vi "OSIPI OPCUA Server Tag Version.vi"(11 "Main Queue Cluster":T62) -> ()   [LabVIEW 2018]
uses:
  <vilib>/OPCUA/controls/NodeId.ctl
  <vilib>/OPCUA/controls/OPC UA Variable Node Refnum.ctl
  <vilib>/OPCUA/controls/OPC UA Server Refnum.ctl
  Drag and Drop/State Cluster.ctl
  support/Message Queue/Message Cluster.ctl
  Drag and Drop/Thumbnail Cluster.ctl
  Drag and Drop/Object Cluster.ctl
  <vilib>/Utility/miscctls.llb/LVRectTypeDef.ctl
  Drag and Drop/Object Type Enum.ctl
  <vilib>/Utility/miscctls.llb/LVPositionTypeDef.ctl
  Config Module/Controls/Main Config Cluster.ctl
  OPC Module Config.ctl
  Scale Module Folder/Measure Instrument/State Enum.ctl
  <vilib>/Utility/miscctls.llb/LVPoint32TypeDef.ctl
  OPC Settings.ctl
  Variable Data Cluster.ctl
  <vilib>/OPCUA/controls/OPC UA StatusCode.ctl
  <vilib>/OPCUA/controls/Subscription ID.ctl
  <vilib>/OPCUA/controls/OPC UA Client Refnum.ctl
  <vilib>/OPCUA/controls/Subscription Data Change.ctl
  <vilib>/OPCUA/controls/Data Type.ctl
  Feed Module/Controls/Feed Module Config Cluster.ctl
  Feed Module/Controls/Feed Module Settings Cluster.ctl
  Ismatec ISM 831C/Controls/Ismatech Settings Cluster.ctl
  Masterflex 7550-30/Controls/Settings Cluster.ctl
  Mettler Toledo/Controls/Settings Cluster.ctl
  Bronkhorst M13 Flow Meter/Settings Cluster.ctl
  Measure Instrument/PID 2 Parameters Cluster.ctl
  Measure Instrument/PID Input Enum.ctl
  Measure Instrument/PID 2 Output Enum.ctl
  Tacmina QI/Tacmina QI DAQ Setting.ctl
  KNF Pump/Settings Cluster plus SIMDOS.ctl
  ASIA Pump/Pump Settings.ctl
  VICI M50 Party Mode/Settings Cluster.ctl
  FLOM Pump/Settings Cluster.ctl
  SSI PR Class/SSI PR Settings Cluster.ctl
  TT Module/Controls/TT Module Config Cluster.ctl
  Acquisition/Hardware Configuration.ctl
  Acquisition/Task Cluster.ctl
  PT Module/Controls/PT Module Config Cluster.ctl
  Scale Module Folder/Feed Module/Controls/Scale Module Config Cluster.ctl
  Scale Module Folder/Feed Module/Controls/Scale Module Settings Cluster.ctl
  Pump Module Folder/Pump Module Config Cluster.ctl
  Pump Module Folder/Pump Module Settings Cluster.ctl
  LabJack Module/Controls/U3 Module Config Cluster.ctl
  Decoration Module/Decoration Module Config Cluster.ctl
  Flow Module Folder/Feed Module/Controls/Flow Module Config Cluster.ctl
  Flow Module Folder/Feed Module/Controls/Flow Module Settings Cluster.ctl
  TCU Module/TCU Module Folder/TCU Module Config Cluster.ctl
  TCU Module/TCU Module Folder/TCU Module Settings Cluster.ctl
  TCU Module/TCU Module Folder/Measure Instrument/Output Devices.ctl
  Huber TCU/Huber Settings.ctl
  Lauda Integral XT-150 TCU/Lauda Settings.ctl
  Julabo Type 1 TCU/Julabo Type 1 TCU Folder/Julabo FP-50 Settings.ctl
  Huber Unistat 410 TCU/Huber Unistat 410 Settings.ctl
  D-O Module Folder/Not Sure Where this is Used.ctl
  Sequencing/Squence Control.ctl
  D-O Module Folder/D-O Module Config Cluster.ctl
  D-O Module Folder/Valve Clusters.ctl
  D-O Module Folder/D-O Module Settings Cluster.ctl
  D-O Module Folder/D-O Device Settings Cluster.ctl
  VICI Electronic Actuator/VICI Electronic Actuator Settings.ctl
  Pressure Regulator Control Module/Pressure Regulator/Controls/4-20mA Module Config Cluster.ctl
  Pressure Regulator Control Module/Pressure Regulator/Controls/4-20mA Module Settings Cluster.ctl
  Pressure Transmitter/Pressure Transmitter Device Settings.ctl
  Pressure Reg Module/Pressure Regulator Device Settings.ctl
  <vilib>/OPCUA/controls/Supported Security Policies.ctl
  Tag VIs/Tag FGV Operation Enum.ctl
  <vilib>/OPCUA/server/Write Double.vi
  <vilib>/OPCUA/NI OPC UA Server.lvlib
  Shared Variables/Dynamic Shared Variables.lvlib
  support/Message Queue/Message Queue.lvlib
  support/Message Queue/Enqueue Message (Single).vi
  TT Module/TT Module.lvlib
  Masterflex 7550-30/Masterflex 7550-30.lvlib
  Ismatec ISM 831C/Ismatec ISM 831C.lvlib
  Tacmina QI/Tacmina QI.lvlib
  KNF Pump/KNF SIMDOS.lvlib
  VICI M50 Party Mode/VICI M6 M50 Party Mode.lvlib
  FLOM Pump/FLOM Pump.lvlib
  ASIA Pump.lvlib
  Mettler Toledo/Mettler Toledo.lvlib
  Bronkhorst M13 Flow Meter/Bronkhorst M13 Flow Meter.lvlib
  SSI PR Class/SSI PR Pump.lvlib
  Feed Module/Feed Module.lvlib
  DAQ/DAQ.lvlib
  PT Module/PT Module.lvlib
  Scale Module Folder/Scale Module.lvlib
  Pump Module Folder/Pump Module.lvlib
  LabJack Module/U3 Module.lvlib
  Flow Module Folder/Flow Module.lvlib
  Huber TCU/Huber Ministat 230 TCU.lvlib
  Lauda Integral XT-150 TCU/Lauda TCU.lvlib
  Julabo Type 1 TCU/Julabo Type 1 TCU Folder/Julabo Type FP-50 TCU.lvlib
  Huber Unistat 410 TCU/Huber Unistat 410 TCU.lvlib
  TCU Module/TCU Module Folder/TCU Module.lvlib
  Sequencing/Sequencing Library.lvlib
  D-O Module Folder/D-O Module.lvlib
  D-O Module Folder/DIO Valve/VICI Electronic Actuator.lvlib
  Pressure Transmitter/Pressure Transmitter Library.lvlib
  Pressure Reg Module/Pressure Regulator Library.lvlib
  Pressure Regulator Control Module/Pressure Regulator/4-20mA Module.lvlib
  OPC UA.lvlib
  Scale Module Folder/Measure Instrument/Scale Module Engine.lvlib
  Config Module/Config Module.lvlib
  Drag and Drop/Drag and Drop.lvlib
panel:
  in  "?":T1={"VI refs"=[], "Queues"=[], "[Thumbnails]"=[], "Drag Object Idx"=0, "[Objects]"=[], "Active Object"=0, "Drop Offset"={"Left"=0, "Top"=0}, "Process Name"="", "Main Config"={"OPC Module Configs"=[], "Feed Module Configs"=[], "Log File Path"=path "", "TT Module Configs"=[], "DAQ Config"={"Tasks"=[]}, "PT Module Configs"=[], "Scale Module Configs"=[], "Pump Module Configs"=[], "U3 Module Configs"=[{"GUID"="", "Drop Coords"={"Horizontal"=0, "Vertical"=0}, "AI Channel Number"=enum."Default", "Process Name"="", "Input Channel Numeric Alarm Settings"=[]}], "Decoration Module Configs"=[], "Flow Module Configs"=[], "TCU Module Configs"=[], "Steps"=[], "Abort"=FALSE, "DO Module Configs"=[], "PR Module Configs"=[], "Cycle Period"=0.0}, "Campaign Filepath"=path "", "Config Changed?"=FALSE} {"Main Config"."PR Module Configs"."Settings"."PID 2 Parameters"."output range"."output low" format="%.2f"; "Main Config"."PR Module Configs"."Settings"."PID 2 Parameters"."output range"."output high" min=0.0 max=100.0 format="%.2f"; "Main Config"."PR Module Configs"."Settings"."PID 2 Parameters"."PID gains"."derivative time (Td, min)" format="%.3f"; "Main Config"."PR Module Configs"."Settings"."PID 2 Parameters"."PID gains"."integral time (Ti, min)" format="%.3f"; "Main Config"."PR Module Configs"."Settings"."PID 2 Parameters"."PID gains"."proportional gain (Kc)" format="%.3f"; "Main Config"."Steps"."Control" items=["Pump %", "Setpoint"]; "Main Config"."TCU Module Configs"."Settings"."Julabo FP-50 Settings"."Pump Power" min=0 max=8 step=1; "Main Config"."TCU Module Configs"."Settings"."Lauda Settings"."Pump Power" min=0 max=8 step=1; "Main Config"."Pump Module Configs"."Settings"."ASIA Pump C"."channel" min=0 max=1 step=1; "Main Config"."Pump Module Configs"."Settings"."Masterflex"."Pump Number" min=1.0 max=20.0 step=1.0; "Main Config"."Pump Module Configs"."Settings"."Ismatech"."Pump Number" min=1.0 max=20.0 step=1.0; "Main Config"."Feed Module Configs"."Settings"."output range"."output low" min=0.0 max=100.0 format="%.2f"; "Main Config"."Feed Module Configs"."Settings"."output range"."output high" format="%.2f"; "Main Config"."Feed Module Configs"."Settings"."PID 2 Parameters"."PID gains"."derivative time (Td, min)" format="%.3f"; "Main Config"."Feed Module Configs"."Settings"."PID 2 Parameters"."PID gains"."integral time (Ti, min)" format="%.3f"; "Main Config"."Feed Module Configs"."Settings"."PID 2 Parameters"."PID gains"."proportional gain (Kc)" format="%.3f"; "Main Config"."Feed Module Configs"."Settings"."ASIA Pump C"."channel" min=0 max=1 step=1; "Main Config"."Feed Module Configs"."Settings"."Ismatech"."Pump Number" min=1.0 max=20.0 step=1.0; "Main Config"."Feed Module Configs"."Settings"."Masterflex"."Pump Number" min=1.0 max=20.0 step=1.0}
  in  "supported security policies (None)":T63={"None"=TRUE, "Sign with Basic128Rsa15"=TRUE, "Sign and Encrypt with Basic128Rsa15"=TRUE, "Sign with Basic256"=TRUE, "Sign and Encrypt with Basic256"=TRUE}
  out "Tag Values":dbl[](array[numeric])
  out "Tag Names":string[](array[string])
  out "Array":T65(array[cluster])
  out "OPC UA server refnum out":T66
  out "Array 2":T14[](array[typedef]) items=["Good"=0, "Good_SubscriptionTransferred"=2949120, "Good_CompletesAsynchronously"=3014656, "Good_Overload"=3080192, "Good_Clamped"=3145728, "Good_LocalOverride"=9830400, "Good_EntryInserted"=10616832, "Good_EntryReplaced"=10682368, "Good_NoData"=10813440, "Good_MoreData"=10878976, "Good_CommunicationEvent"=10944512, "Good_ShutdownEvent"=11010048, "Good_CallAgain"=11075584, "Good_NonCriticalTimeout"=11141120, "Good_ResultsMayBeIncomplete"=12189696, "Good_DataIgnored"=14221312, "Uncertain"=1073741824, "Uncertain_ReferenceOutOfServer"=1080819712, "Uncertain_NoCommunicationLastUsableValue"=1083113472, "Uncertain_LastUsableValue"=1083179008, "Uncertain_SubstituteValue"=1083244544, "Uncertain_InitialValue"=1083310080, "Uncertain_SensorNotAccurate"=1083375616, "Uncertain_EngineeringUnitsExceeded"=1083441152, "Uncertain_SubNormal"=1083506688, "Uncertain_DataSubNormal"=1084489728, "Uncertain_ReferenceNotDeleted"=1086062592, "Uncertain_NotAllNodesAvailable"=1086324736, "Bad"=2147483648, "Bad_UnexpectedError"=2147549184, "Bad_InternalError"=2147614720, "Bad_OutOfMemory"=2147680256, "Bad_ResourceUnavailable"=2147745792, "Bad_CommunicationError"=2147811328, "Bad_EncodingError"=2147876864, "Bad_DecodingError"=2147942400, "Bad_EncodingLimitsExceeded"=2148007936, "Bad_UnknownResponse"=2148073472, "Bad_Timeout"=2148139008, "Bad_ServiceUnsupported"=2148204544, "Bad_Shutdown"=2148270080, "Bad_ServerNotConnected"=2148335616, "Bad_ServerHalted"=2148401152, "Bad_NothingToDo"=2148466688, "Bad_TooManyOperations"=2148532224, "Bad_DataTypeIdUnknown"=2148597760, "Bad_CertificateInvalid"=2148663296, "Bad_SecurityChecksFailed"=2148728832, "Bad_CertificateTimeInvalid"=2148794368, "Bad_CertificateIssuerTimeInvalid"=2148859904, "Bad_CertificateHostNameInvalid"=2148925440, "Bad_CertificateUriInvalid"=2148990976, "Bad_CertificateUseNotAllowed"=2149056512, "Bad_CertificateIssuerUseNotAllowed"=2149122048, "Bad_CertificateUntrusted"=2149187584, "Bad_CertificateRevocationUnknown"=2149253120, "Bad_CertificateIssuerRevocationUnknown"=2149318656, "Bad_CertificateRevoked"=2149384192, "Bad_CertificateIssuerRevoked"=2149449728, "Bad_UserAccessDenied"=2149515264, "Bad_IdentityTokenInvalid"=2149580800, "Bad_IdentityTokenRejected"=2149646336, "Bad_SecureChannelIdInvalid"=2149711872, "Bad_InvalidTimestamp"=2149777408, "Bad_NonceInvalid"=2149842944, "Bad_SessionIdInvalid"=2149908480, "Bad_SessionClosed"=2149974016, "Bad_SessionNotActivated"=2150039552, "Bad_SubscriptionIdInvalid"=2150105088, "Bad_RequestHeaderInvalid"=2150236160, "Bad_TimestampsToReturnInvalid"=2150301696, "Bad_RequestCancelledByClient"=2150367232, "Bad_NoCommunication"=2150694912, "Bad_WaitingForInitialData"=2150760448, "Bad_NodeIdInvalid"=2150825984, "Bad_NodeIdUnknown"=2150891520, "Bad_AttributeIdInvalid"=2150957056, "Bad_IndexRangeInvalid"=2151022592, "Bad_IndexRangeNoData"=2151088128, "Bad_DataEncodingInvalid"=2151153664, "Bad_DataEncodingUnsupported"=2151219200, "Bad_NotReadable"=2151284736, "Bad_NotWritable"=2151350272, "Bad_OutOfRange"=2151415808, "Bad_NotSupported"=2151481344, "Bad_NotFound"=2151546880, "Bad_ObjectDeleted"=2151612416, "Bad_NotImplemented"=2151677952, "Bad_MonitoringModeInvalid"=2151743488, "Bad_MonitoredItemIdInvalid"=2151809024, "Bad_MonitoredItemFilterInvalid"=2151874560, "Bad_MonitoredItemFilterUnsupported"=2151940096, "Bad_FilterNotAllowed"=2152005632, "Bad_StructureMissing"=2152071168, "Bad_EventFilterInvalid"=2152136704, "Bad_ContentFilterInvalid"=2152202240, "Bad_FilterOperandInvalid"=2152267776, "Bad_ContinuationPointInvalid"=2152333312, "Bad_NoContinuationPoints"=2152398848, "Bad_ReferenceTypeIdInvalid"=2152464384, "Bad_BrowseDirectionInvalid"=2152529920, "Bad_NodeNotInView"=2152595456, "Bad_ServerUriInvalid"=2152660992, "Bad_ServerNameMissing"=2152726528, "Bad_DiscoveryUrlMissing"=2152792064, "Bad_SempahoreFileMissing"=2152857600, "Bad_RequestTypeInvalid"=2152923136, "Bad_SecurityModeRejected"=2152988672, "Bad_SecurityPolicyRejected"=2153054208, "Bad_TooManySessions"=2153119744, "Bad_UserSignatureInvalid"=2153185280, "Bad_ApplicationSignatureInvalid"=2153250816, "Bad_NoValidCertificates"=2153316352, "Bad_RequestCancelledByRequest"=2153381888, "Bad_ParentNodeIdInvalid"=2153447424, "Bad_ReferenceNotAllowed"=2153512960, "Bad_NodeIdRejected"=2153578496, "Bad_NodeIdExists"=2153644032, "Bad_NodeClassInvalid"=2153709568, "Bad_BrowseNameInvalid"=2153775104, "Bad_BrowseNameDuplicated"=2153840640, "Bad_NodeAttributesInvalid"=2153906176, "Bad_TypeDefinitionInvalid"=2153971712, "Bad_SourceNodeIdInvalid"=2154037248, "Bad_TargetNodeIdInvalid"=2154102784, "Bad_DuplicateReferenceNotAllowed"=2154168320, "Bad_InvalidSelfReference"=2154233856, "Bad_ReferenceLocalOnly"=2154299392, "Bad_NoDeleteRights"=2154364928, "Bad_ServerIndexInvalid"=2154430464, "Bad_ViewIdUnknown"=2154496000, "Bad_TooManyMatches"=2154627072, "Bad_QueryTooComplex"=2154692608, "Bad_NoMatch"=2154758144, "Bad_MaxAgeInvalid"=2154823680, "Bad_HistoryOperationInvalid"=2154889216, "Bad_HistoryOperationUnsupported"=2154954752, "Bad_WriteNotSupported"=2155020288, "Bad_TypeMismatch"=2155085824, "Bad_MethodInvalid"=2155151360, "Bad_ArgumentsMissing"=2155216896, "Bad_TooManySubscriptions"=2155282432, "Bad_TooManyPublishRequests"=2155347968, "Bad_NoSubscription"=2155413504, "Bad_SequenceNumberUnknown"=2155479040, "Bad_MessageNotAvailable"=2155544576, "Bad_InsufficientClientProfile"=2155610112, "Bad_TcpServerTooBusy"=2155675648, "Bad_TcpMessageTypeInvalid"=2155741184, "Bad_TcpSecureChannelUnknown"=2155806720, "Bad_TcpMessageTooLarge"=2155872256, "Bad_TcpNotEnoughResources"=2155937792, "Bad_TcpInternalError"=2156003328, "Bad_TcpEndpointUrlInvalid"=2156068864, "Bad_RequestInterrupted"=2156134400, "Bad_RequestTimeout"=2156199936, "Bad_SecureChannelClosed"=2156265472, "Bad_SecureChannelTokenUnknown"=2156331008, "Bad_SequenceNumberInvalid"=2156396544, "Bad_ConfigurationError"=2156462080, "Bad_NotConnected"=2156527616, "Bad_DeviceFailure"=2156593152, "Bad_SensorFailure"=2156658688, "Bad_OutOfService"=2156724224, "Bad_DeadbandFilterInvalid"=2156789760, "Bad_RefreshInProgress"=2157379584, "Bad_ConditionAlreadyDisabled"=2157445120, "Bad_ConditionDisabled"=2157510656, "Bad_EventIdUnknown"=2157576192, "Bad_NoData"=2157641728, "Bad_DataLost"=2157772800, "Bad_DataUnavailable"=2157838336, "Bad_EntryExists"=2157903872, "Bad_NoEntryExists"=2157969408, "Bad_TimestampNotSupported"=2158034944, "Bad_InvalidArgument"=2158690304, "Bad_ConnectionRejected"=2158755840, "Bad_Disconnect"=2158821376, "Bad_ConnectionClosed"=2158886912, "Bad_InvalidState"=2158952448, "Bad_EndOfStream"=2159017984, "Bad_NoDataAvailable"=2159083520, "Bad_WaitingForResponse"=2159149056, "Bad_OperationAbandoned"=2159214592, "Bad_ExpectedStreamToBlock"=2159280128, "Bad_WouldBlock"=2159345664, "Bad_SyntaxError"=2159411200, "Bad_MaxConnectionsReached"=2159476736, "Bad_RequestTooLarge"=2159542272, "Bad_ResponseTooLarge"=2159607808, "Bad_EventNotAcknowledgeable"=2159738880, "Bad_InvalidTimestampArgument"=2159869952, "Bad_ProtocolVersionUnsupported"=2159935488, "Bad_StateNotActive"=2160001024, "Bad_FilterOperatorInvalid"=2160132096, "Bad_FilterOperatorUnsupported"=2160197632, "Bad_FilterOperandCountMismatch"=2160263168, "Bad_FilterElementInvalid"=2160328704, "Bad_FilterLiteralInvalid"=2160394240, "Bad_IdentityChangeNotSupported"=2160459776, "Bad_NotTypeDefinition"=2160590848, "Bad_ViewTimestampInvalid"=2160656384, "Bad_ViewParameterMismatch"=2160721920, "Bad_ViewVersionInvalid"=2160787456, "Bad_ConditionAlreadyEnabled"=2160852992, "Bad_DialogNotActive"=2160918528, "Bad_DialogResponseInvalid"=2160984064, "Bad_ConditionBranchAlreadyAcked"=2161049600, "Bad_ConditionBranchAlreadyConfirmed"=2161115136, "Bad_ConditionAlreadyShelved"=2161180672, "Bad_ConditionNotShelved"=2161246208, "Bad_ShelvingTimeOutOfRange"=2161311744, "Bad_AggregateListMismatch"=2161377280, "Bad_AggregateNotSupported"=2161442816, "Bad_AggregateInvalidInputs"=2161508352, "Bad_BoundNotFound"=2161573888, "Bad_BoundNotSupported"=2161639424, "Bad_AggregateConfigurationRejected"=2161770496, "Bad_TooManyMonitoredItems"=2161836032]
  out "server endpoint URL":string
  in  "?":T1 {"Main Config"."PR Module Configs"."Settings"."PID 2 Parameters"."output range"."output low" format="%.2f"; "Main Config"."PR Module Configs"."Settings"."PID 2 Parameters"."output range"."output high" min=0.0 max=100.0 format="%.2f"; "Main Config"."PR Module Configs"."Settings"."PID 2 Parameters"."PID gains"."derivative time (Td, min)" format="%.3f"; "Main Config"."PR Module Configs"."Settings"."PID 2 Parameters"."PID gains"."integral time (Ti, min)" format="%.3f"; "Main Config"."PR Module Configs"."Settings"."PID 2 Parameters"."PID gains"."proportional gain (Kc)" format="%.3f"; "Main Config"."Steps"."Control" items=["Pump %", "Setpoint"]; "Main Config"."TCU Module Configs"."Settings"."Julabo FP-50 Settings"."Pump Power" min=0 max=8 step=1; "Main Config"."TCU Module Configs"."Settings"."Lauda Settings"."Pump Power" min=0 max=8 step=1; "Main Config"."Pump Module Configs"."Settings"."ASIA Pump C"."channel" min=0 max=1 step=1; "Main Config"."Pump Module Configs"."Settings"."Masterflex"."Pump Number" min=1.0 max=20.0 step=1.0; "Main Config"."Pump Module Configs"."Settings"."Ismatech"."Pump Number" min=1.0 max=20.0 step=1.0; "Main Config"."Feed Module Configs"."Settings"."output range"."output low" min=0.0 max=100.0 format="%.2f"; "Main Config"."Feed Module Configs"."Settings"."output range"."output high" format="%.2f"; "Main Config"."Feed Module Configs"."Settings"."PID 2 Parameters"."PID gains"."derivative time (Td, min)" format="%.3f"; "Main Config"."Feed Module Configs"."Settings"."PID 2 Parameters"."PID gains"."integral time (Ti, min)" format="%.3f"; "Main Config"."Feed Module Configs"."Settings"."PID 2 Parameters"."PID gains"."proportional gain (Kc)" format="%.3f"; "Main Config"."Feed Module Configs"."Settings"."ASIA Pump C"."channel" min=0 max=1 step=1; "Main Config"."Feed Module Configs"."Settings"."Ismatech"."Pump Number" min=1.0 max=20.0 step=1.0; "Main Config"."Feed Module Configs"."Settings"."Masterflex"."Pump Number" min=1.0 max=20.0 step=1.0}
  out "OPC UA server refnum out 3":T66
  out "Array 3":T65(array[cluster])
  # "Instrument Settings"
  # "Instrument Settings"
  # "Output Instruments"
  # "Flow Meter Settings"
  # "Output Instruments"
  # "Scale Settings"
  # "Output Instruments"
  # "Input Instruments"
  # "Instrument Settings"
  # "Instrument Settings"
  # "Output Instruments"
  # "Flow Meter Settings"
  # "Output Instruments"
  # "Scale Settings"
  # "Output Instruments"
  # "Input Instruments"
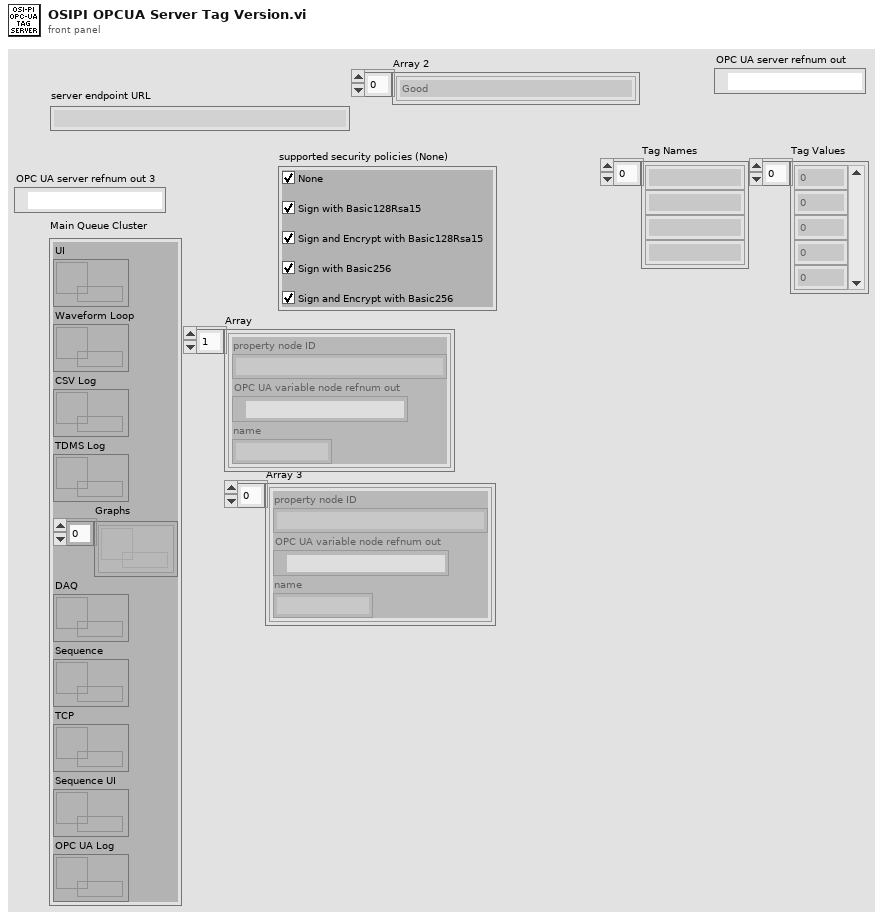
[diagram p1: front panel]
types:
  T1 = typedef "Drag and Drop.lvlib/State Cluster.ctl" = cluster{"VI refs":refnum<vi>[], "Queues":refnum<queue>[], "[Thumbnails]":T2[], "Drag Object Idx":i32, "[Objects]":T3[], "Active Object":i32, "Drop Offset":T6, "Process Name":string, "Main Config":T7, "Campaign Filepath":path, "Config Changed?":bool}
  T2 = typedef "Thumbnail Cluster.ctl" = cluster{"Path":path, "Rectangle":cluster{"left":i16, "top":i16, "right":i16, "bottom":i16}}
  T3 = typedef "Object Cluster.ctl" = cluster{"BMP Path":path, "Anchor Position":cluster{"X":i32, "Y":i32}, "Hot Spot":T4, "Type":T5, "Parameters":variant}
  T4 = typedef "LVRectTypeDef.ctl" = cluster{"Left":i16, "Top":i16, "Right":i16, "Bottom":i16}
  T5 = typedef "Object Type Enum.ctl" = enum16{"Icon", "Line", "Text", "Feed Module"}
  T6 = typedef "LVPositionTypeDef.ctl" = cluster{"Left":i32, "Top":i32}
  T7 = typedef "Config Module.lvlib/Main Config Cluster.ctl" = cluster{"OPC Module Configs":T8[], "Feed Module Configs":T17[], "Log File Path":path, "TT Module Configs":T32[], "DAQ Config":T33, "PT Module Configs":T35[], "Scale Module Configs":T36[], "Pump Module Configs":T38[], "U3 Module Configs":T40[], "Decoration Module Configs":T41[], "Flow Module Configs":T42[], "TCU Module Configs":T44[], "Steps":T51, "Abort":bool, "DO Module Configs":T53[], "PR Module Configs":T58[], "Cycle Period":dbl}
  T8 = typedef "OPC UA.lvlib/OPC Module Config.ctl" = cluster{"State":T9, "GUID":string, "Drop Coords":T10, "Configuration":T11, "First Iteration":bool, "Data":cluster{"Object Name":string, "Variable Array":T12[]}[], "Process Name":string, "Load Count":i32, "Log Started":bool, "subscription ID out":T15, "OPC UA client refnum out":T16, "Event Registration Refnum":refnum<event-registration>, "Start Time":timestamp, "Current Time":timestamp}
  T9 = typedef "Scale Module.lvlib/Scale Module Engine.lvlib/State Enum.ctl" = enum16{"Measuring", "Idle"}
  T10 = typedef "LVPoint32TypeDef.ctl" = cluster{"Horizontal":i32, "Vertical":i32}
  T11 = typedef "OPC UA.lvlib/OPC Settings.ctl" = cluster{"Cycle Period":dbl, "server endpoint URL":string, "security policy":cluster{"message mode":enum16{"None", "Sign", "Sign and Encrypt"}, "security":enum16{"Basic256", "Basic128Rsa15"}}, "Trust Any Server":bool}
  T12 = typedef "OPC UA.lvlib/Variable Data Cluster.ctl" = cluster{"node ID":T13, "browse name":string, "status":T14, "timestamp":timestamp, "value ":variant}
  T13 = typedef "NodeId.ctl" = string
  T14 = typedef "OPC UA StatusCode.ctl" = u32
  T15 = typedef "Subscription ID.ctl" = u32
  T16 = typedef "OPC UA Client Refnum.ctl" = refnum<k21>
  T17 = typedef "Feed Module.lvlib/Feed Module Config Cluster.ctl" = cluster{"GUID":string, "Drop Coords":T10, "Process Name":string, "Settings":T18, "Settings Load Count":i32, "OP Load Count":i32}
  T18 = typedef "Feed Module.lvlib/Feed Module Settings Cluster.ctl" = cluster{"Cycle Period":dbl, "Ismatech":T19, "Masterflex":T20, "Mettler":T21, "Bronkhorst M13 Flow Meter":T22, "PID 2 Parameters":T23, "Manual Entry":dbl, "Auto?":bool, "output range":cluster{"output high":dbl, "output low":dbl}, "Bronkhorst M14":T21, "Tacmina Settings":T26, "KNF SIMDOS Settings":T27, "ASIA Pump C":T28, "VICI Settings":T29, "FLOM Settings":T30, "SSI PR Settings":T31}
  T19 = typedef "Ismatec ISM 831C.lvlib/Ismatech Settings Cluster.ctl" = cluster{"VISA resource name":refnum<visa-resource-name>, "Simulated?":bool, "Pump Number":dbl, "Reverse?":bool}
  T20 = typedef "Masterflex 7550-30.lvlib/Settings Cluster.ctl" = cluster{"VISA resource name":refnum<visa-resource-name>, "Simulated?":bool, "Pump Number":dbl, "Reverse?":bool}
  T21 = typedef "Mettler Toledo.lvlib/Settings Cluster.ctl" = cluster{"VISA resource name":refnum<visa-resource-name>, "Simulated?":bool}
  T22 = typedef "Bronkhorst M13 Flow Meter.lvlib/Settings Cluster.ctl" = cluster{"VISA resource name":refnum<visa-resource-name>, "Simulated?":bool}
  T23 = typedef "PID 2 Parameters Cluster.ctl" = cluster{"Input Device":T24, "Output Device":T25, "Setpoint":dbl, "PID gains":cluster{"proportional gain (Kc)":dbl, "integral time (Ti, min)":dbl, "derivative time (Td, min)":dbl}}
  T24 = typedef "PID Input Enum.ctl" = enum16{"Default", "Bronkhorst M13", "Bronkhorst M14", "Scale Rate of Change"}
  T25 = typedef "PID 2 Output Enum.ctl" = enum16{"Default", "Ismatec ISM 831C", "Masterflex 7550-30", "VICI", "Tacmina QI", "KNF SIMDOS", "ASIA Type C", "FLOM UI-22-11", "SSI PR"}
  T26 = typedef "Tacmina QI.lvlib/Tacmina QI DAQ Setting.ctl" = cluster{"Analog DAQ Task":refnum<k21>, "Digital DAQ Task":refnum<k21>}
  T27 = typedef "KNF SIMDOS.lvlib/Settings Cluster plus SIMDOS.ctl" = cluster{"VISA resource name":refnum<visa-resource-name>, "Simulated?":bool}
  T28 = typedef "ASIA Pump.lvlib/Pump Settings.ctl" = cluster{"ASIA Pump #":i32, "channel":i32, "Simulated":bool}
  T29 = typedef "VICI M6 M50 Party Mode.lvlib/Settings Cluster.ctl" = cluster{"VISA resource name":refnum<visa-resource-name>, "Simulated?":bool, "Pump Letter":string, "Reverse?":bool}
  T30 = typedef "FLOM Pump.lvlib/Settings Cluster.ctl" = cluster{"VISA resource name":refnum<visa-resource-name>, "Simulated?":bool, "Pump Number":dbl}
  T31 = typedef "SSI PR Pump.lvlib/SSI PR Settings Cluster.ctl" = cluster{"VISA resource name":refnum<visa-resource-name>, "Simulated?":bool}
  T32 = typedef "TT Module.lvlib/TT Module Config Cluster.ctl" = cluster{"GUID":string, "Drop Coords":T10, "Input Channel Tag Name ":string, "Process Name":string, "Input Channel Numeric Alarm Settings":cluster{"enable? (F)":bool, "name":string, "alarm type":enum16{"HI_HI", "HI", "LO", "LO_LO"}, "level/change":dbl, "deadband/time":dbl, "priority":u32, "ack type":enum16{"Auto", "User", "None", "Each Occurrence"}, "area":string, "description":string, "log? (T)":bool}[]}
  T33 = typedef "DAQ.lvlib/Hardware Configuration.ctl" = cluster{"Tasks":T34[]}
  T34 = typedef "Task Cluster.ctl" = cluster{"DAQmx Task":refnum<k21>, "Read-Write Radio":enum32{"Read", "Write"}}
  T35 = typedef "PT Module.lvlib/PT Module Config Cluster.ctl" = cluster{"GUID":string, "Drop Coords":T10, "Input Channel Tag Name ":string, "Process Name":string, "Input Channel Numeric Alarm Settings":cluster{"enable? (F)":bool, "name":string, "alarm type":enum16{"HI_HI", "HI", "LO", "LO_LO"}, "level/change":dbl, "deadband/time":dbl, "priority":u32, "ack type":enum16{"Auto", "User", "None", "Each Occurrence"}, "area":string, "description":string, "log? (T)":bool}[]}
  T36 = typedef "Scale Module.lvlib/Scale Module Config Cluster.ctl" = cluster{"GUID":string, "Drop Coords":T10, "Process Name":string, "Settings":T37, "Load Count":i32}
  T37 = typedef "Scale Module.lvlib/Scale Module Settings Cluster.ctl" = cluster{"Cycle Period":dbl, "Mettler":T21, "Scale Type":string}
  T38 = typedef "Pump Module.lvlib/Pump Module Config Cluster.ctl" = cluster{"GUID":string, "Drop Coords":T10, "Process Name":string, "Settings":T39, "Load Count":i32}
  T39 = typedef "Pump Module.lvlib/Pump Module Settings Cluster.ctl" = cluster{"Cycle Period":dbl, "Ismatech":T19, "Masterflex":T20, "Manual Entry":dbl, "VICI Settings":T29, "Output Device":T25, "Tacmina Settings":T26, "KNF SIMDOS Settings":T27, "ASIA Pump C":T28, "FLOM Settings":T30, "Pump Calibration File":path, "Calibration":dbl, "Pump Cal Enum":u16, "SSI PR Settings":T31}
  T40 = typedef "U3 Module.lvlib/U3 Module Config Cluster.ctl" = cluster{"GUID":string, "Drop Coords":T10, "AI Channel Number":enum16{"Default", "AI0", "AI1", "AI2", "AI3", "AI4", "AI5", "AI6", "AI7"}, "Process Name":string, "Input Channel Numeric Alarm Settings":cluster{"enable? (F)":bool, "name":string, "alarm type":enum16{"HI_HI", "HI", "LO", "LO_LO"}, "level/change":dbl, "deadband/time":dbl, "priority":u32, "ack type":enum16{"Auto", "User", "None", "Each Occurrence"}, "area":string, "description":string, "log? (T)":bool}[]}
  T41 = typedef "Decoration Module Config Cluster.ctl" = cluster{"GUID":string, "Drop Coords":T10, "Decoration Filepath":path}
  T42 = typedef "Flow Module.lvlib/Flow Module Config Cluster.ctl" = cluster{"GUID":string, "Drop Coords":T10, "Process Name":string, "Settings":T43, "Load Count":i32}
  T43 = typedef "Flow Module.lvlib/Flow Module Settings Cluster.ctl" = cluster{"Cycle Period":dbl, "Bronkhorst M13":T21, "Flow Meter Type":string, "Bronkhorst M14":T21}
  T44 = typedef "TCU Module.lvlib/TCU Module Config Cluster.ctl" = cluster{"GUID":string, "Drop Coords":T10, "Process Name":string, "Settings":T45, "Load Count":i32, "Power Level Changed":bool}
  T45 = typedef "TCU Module.lvlib/TCU Module Settings Cluster.ctl" = cluster{"Cycle Period":dbl, "Setpoint Entry":dbl, "Output Device":T46, "Huber Ministat 230 Settings":T47, "Lauda Settings":T48, "Julabo FP-50 Settings":T49, "Internal Control?":bool, "Huber Unistat 410 Settings":T50}
  T46 = typedef "Output Devices.ctl" = enum16{"Default", "Huber Ministat 230", "Huber Unistat 410", "Lauda XT-150", "Julabo FP-50"}
  T47 = typedef "Huber Ministat 230 TCU.lvlib/Huber Settings.ctl" = cluster{"VISA resource name":refnum<visa-resource-name>, "Simulated?":bool}
  T48 = typedef "Lauda TCU.lvlib/Lauda Settings.ctl" = cluster{"VISA resource name":refnum<visa-resource-name>, "Simulated?":bool, "Pump Power":i32}
  T49 = typedef "Julabo Type FP-50 TCU.lvlib/Julabo FP-50 Settings.ctl" = cluster{"VISA resource name":refnum<visa-resource-name>, "Simulated?":bool, "Pump Power":i32}
  T50 = typedef "Huber Unistat 410 TCU.lvlib/Huber Unistat 410 Settings.ctl" = cluster{"VISA resource name":refnum<visa-resource-name>, "Simulated?":bool}
  T51 = typedef "Not Sure Where this is Used.ctl" = T52[]
  T52 = typedef "Sequencing Library.lvlib/Squence Control.ctl" = cluster{"Module":string, "Control":u16, "Value":dbl, "Wait (sec)":dbl}
  T53 = typedef "D-O Module.lvlib/D-O Module Config Cluster.ctl" = cluster{"GUID":string, "Drop Coords":T10, "Process Name":string, "Settings":T54, "Load Count":i32}
  T54 = typedef "D-O Module.lvlib/Valve Clusters.ctl" = cluster{"Valve Settings":T55, "Valve Type":enum16{"Default", "Digital Output Valve", "VICI Electronic Actuator"}, "Time On (Sec)":dbl, "Time Off (Sec)":dbl, "Run?":bool}
  T55 = typedef "D-O Module.lvlib/D-O Module Settings Cluster.ctl" = cluster{"D-O Settings":T56, "VICI Electronic Actuator":T57}
  T56 = typedef "D-O Module.lvlib/D-O Device Settings Cluster.ctl" = cluster{"DAQmx Task Name":refnum<k21>, "Output Channel":u16, "Output Channel Names":string[]}
  T57 = typedef "VICI Electronic Actuator.lvlib/VICI Electronic Actuator Settings.ctl" = cluster{"VISA resource name":refnum<visa-resource-name>, "Mode":enum16{"Two Positions With Stops", "Two Positions Without Stops", "Mutiposition"}, "Simulated":bool}
  T58 = typedef "4-20mA Module.lvlib/4-20mA Module Config Cluster.ctl" = cluster{"GUID":string, "Drop Coords":T10, "Process Name":string, "Settings":T59, "Settings Load Count":i32}
  T59 = typedef "4-20mA Module.lvlib/4-20mA Module Settings Cluster.ctl" = cluster{"Cycle Period":dbl, "PID 2 Parameters":cluster{"Input Device":enum16{"Default", "4-20mA"}, "Output Device":enum16{"Default", "Equilibar Pressure Reg", "Flow Regulator"}, "Setpoint":dbl, "PID gains":cluster{"proportional gain (Kc)":dbl, "integral time (Ti, min)":dbl, "derivative time (Td, min)":dbl}, "output range":cluster{"output low":dbl, "output high":dbl}}, "Manual Entry":dbl, "Auto?":bool, "4-20mA Input Settings":T60, "4-20mA Out Settings":T61, "Input Channel Tag Name ":string}
  T60 = typedef "Pressure Transmitter Library.lvlib/Pressure Transmitter Device Settings.ctl" = cluster{"Input Channel ":u16}
  T61 = typedef "Pressure Regulator Library.lvlib/Pressure Regulator Device Settings.ctl" = cluster{"Output DAQ Task":refnum<k21>}
  T62 = cluster{"UI":refnum<queue>, "Waveform Loop":refnum<queue>, "CSV Log":refnum<queue>, "TDMS Log":refnum<queue>, "Graphs":refnum<queue>[], "DAQ":refnum<queue>, "Sequence":refnum<queue>, "TCP":refnum<queue>, "Sequence UI":refnum<queue>, "OPC UA Log":refnum<queue>}
  T63 = typedef "Supported Security Policies.ctl" = cluster{"None":bool, "Sign with Basic128Rsa15":bool, "Sign and Encrypt with Basic128Rsa15":bool, "Sign with Basic256":bool, "Sign and Encrypt with Basic256":bool}
  T64 = typedef "OPC UA Variable Node Refnum.ctl" = refnum<k21>
  T65 = cluster{"property node ID":T13, "OPC UA variable node refnum out":T64, "name":string}[]
  T66 = typedef "OPC UA Server Refnum.ctl" = refnum<k21>
  T67 = cluster{"property node ID":T13, "OPC UA variable node refnum out":T64, "name":string}
  T68 = typedef "Data Type.ctl" = u16
  T69 = cluster{"name":string, "data type":T68, "access level":u16, "description":string}
  T70 = typedef "Tag FGV Operation Enum.ctl" = enum16{"Init", "Set Notification Queue", "Create Tag", "Commit", "Write Tag (Numeric)", "Write Tag (Boolean)", "Read All Tags", "Read One Tag", "Delete Tag Category", "Set Alarm Parameters (Numeric)", "Set Alarm Parameters (Boolean)", "Enable All Alarms", "Disable All Alarms", "Delete All Tags", "Read Alarms", "Ack Alarm"}
  T71 = typedef "Feed Module.lvlib/Feed Module Tag Names Cluster.ctl" = cluster{"Pump Flow Tag":string, "PID 2 Out Tag":string, "Scale Tag":string, "Density Tag":string, "FL Temp":string, "Input Device Tag":string, "Output Device Tag":string, "Pump's Flow":string, "Pump's Pressure":string, "Overpressure Tag":string}
  T72 = typedef "Pump Module.lvlib/Pump Module Tag Names Cluster.ctl" = cluster{"Pump Speed":string, "Pump Flow":string, "Pump Pressure":string, "Output Device Tag":string, "Overpressure Tag":string}
  T73 = typedef "Flow Module.lvlib/Tag Cluster.ctl" = cluster{"Flow Tag":string, "Input Disconnected":string, "Density Tag":string, "Temp Tag":string}
  T74 = typedef "TCU Module.lvlib/TCU Module Tag Names Cluster.ctl" = cluster{"TCU Temp":string, "Output Device Tag":string, "TCU Speed":string}
  T75 = typedef "4-20mA Module.lvlib/4-20mA Module Tag Names Cluster.ctl" = cluster{"4-20mA Input":string, "PID 2 Out Tag":string, "4-20mA Output":string, "Input Device Tag":string, "Output Device Tag":string}
  T76 = cluster{"Feed Module Tags Array":T71[], "DAQ Tags Array":string[], "Scale Tags Array":cluster{"Scale Value":string, "Scale Error":string}[], "Pump Module Tags Array":T72[], "Flow Module Tags Array":T73[], "TCU Module Tags Array":T74[], "PR Module Tags Array":T75[], "OPC Module Tags Array":cluster{"OPC UA Error":string, "Array of Names":string[]}[]}
  T77 = cluster{"Scale Value":string, "Scale Error":string}[]
  T78 = cluster{"OPC UA Error":string, "Array of Names":string[]}[]
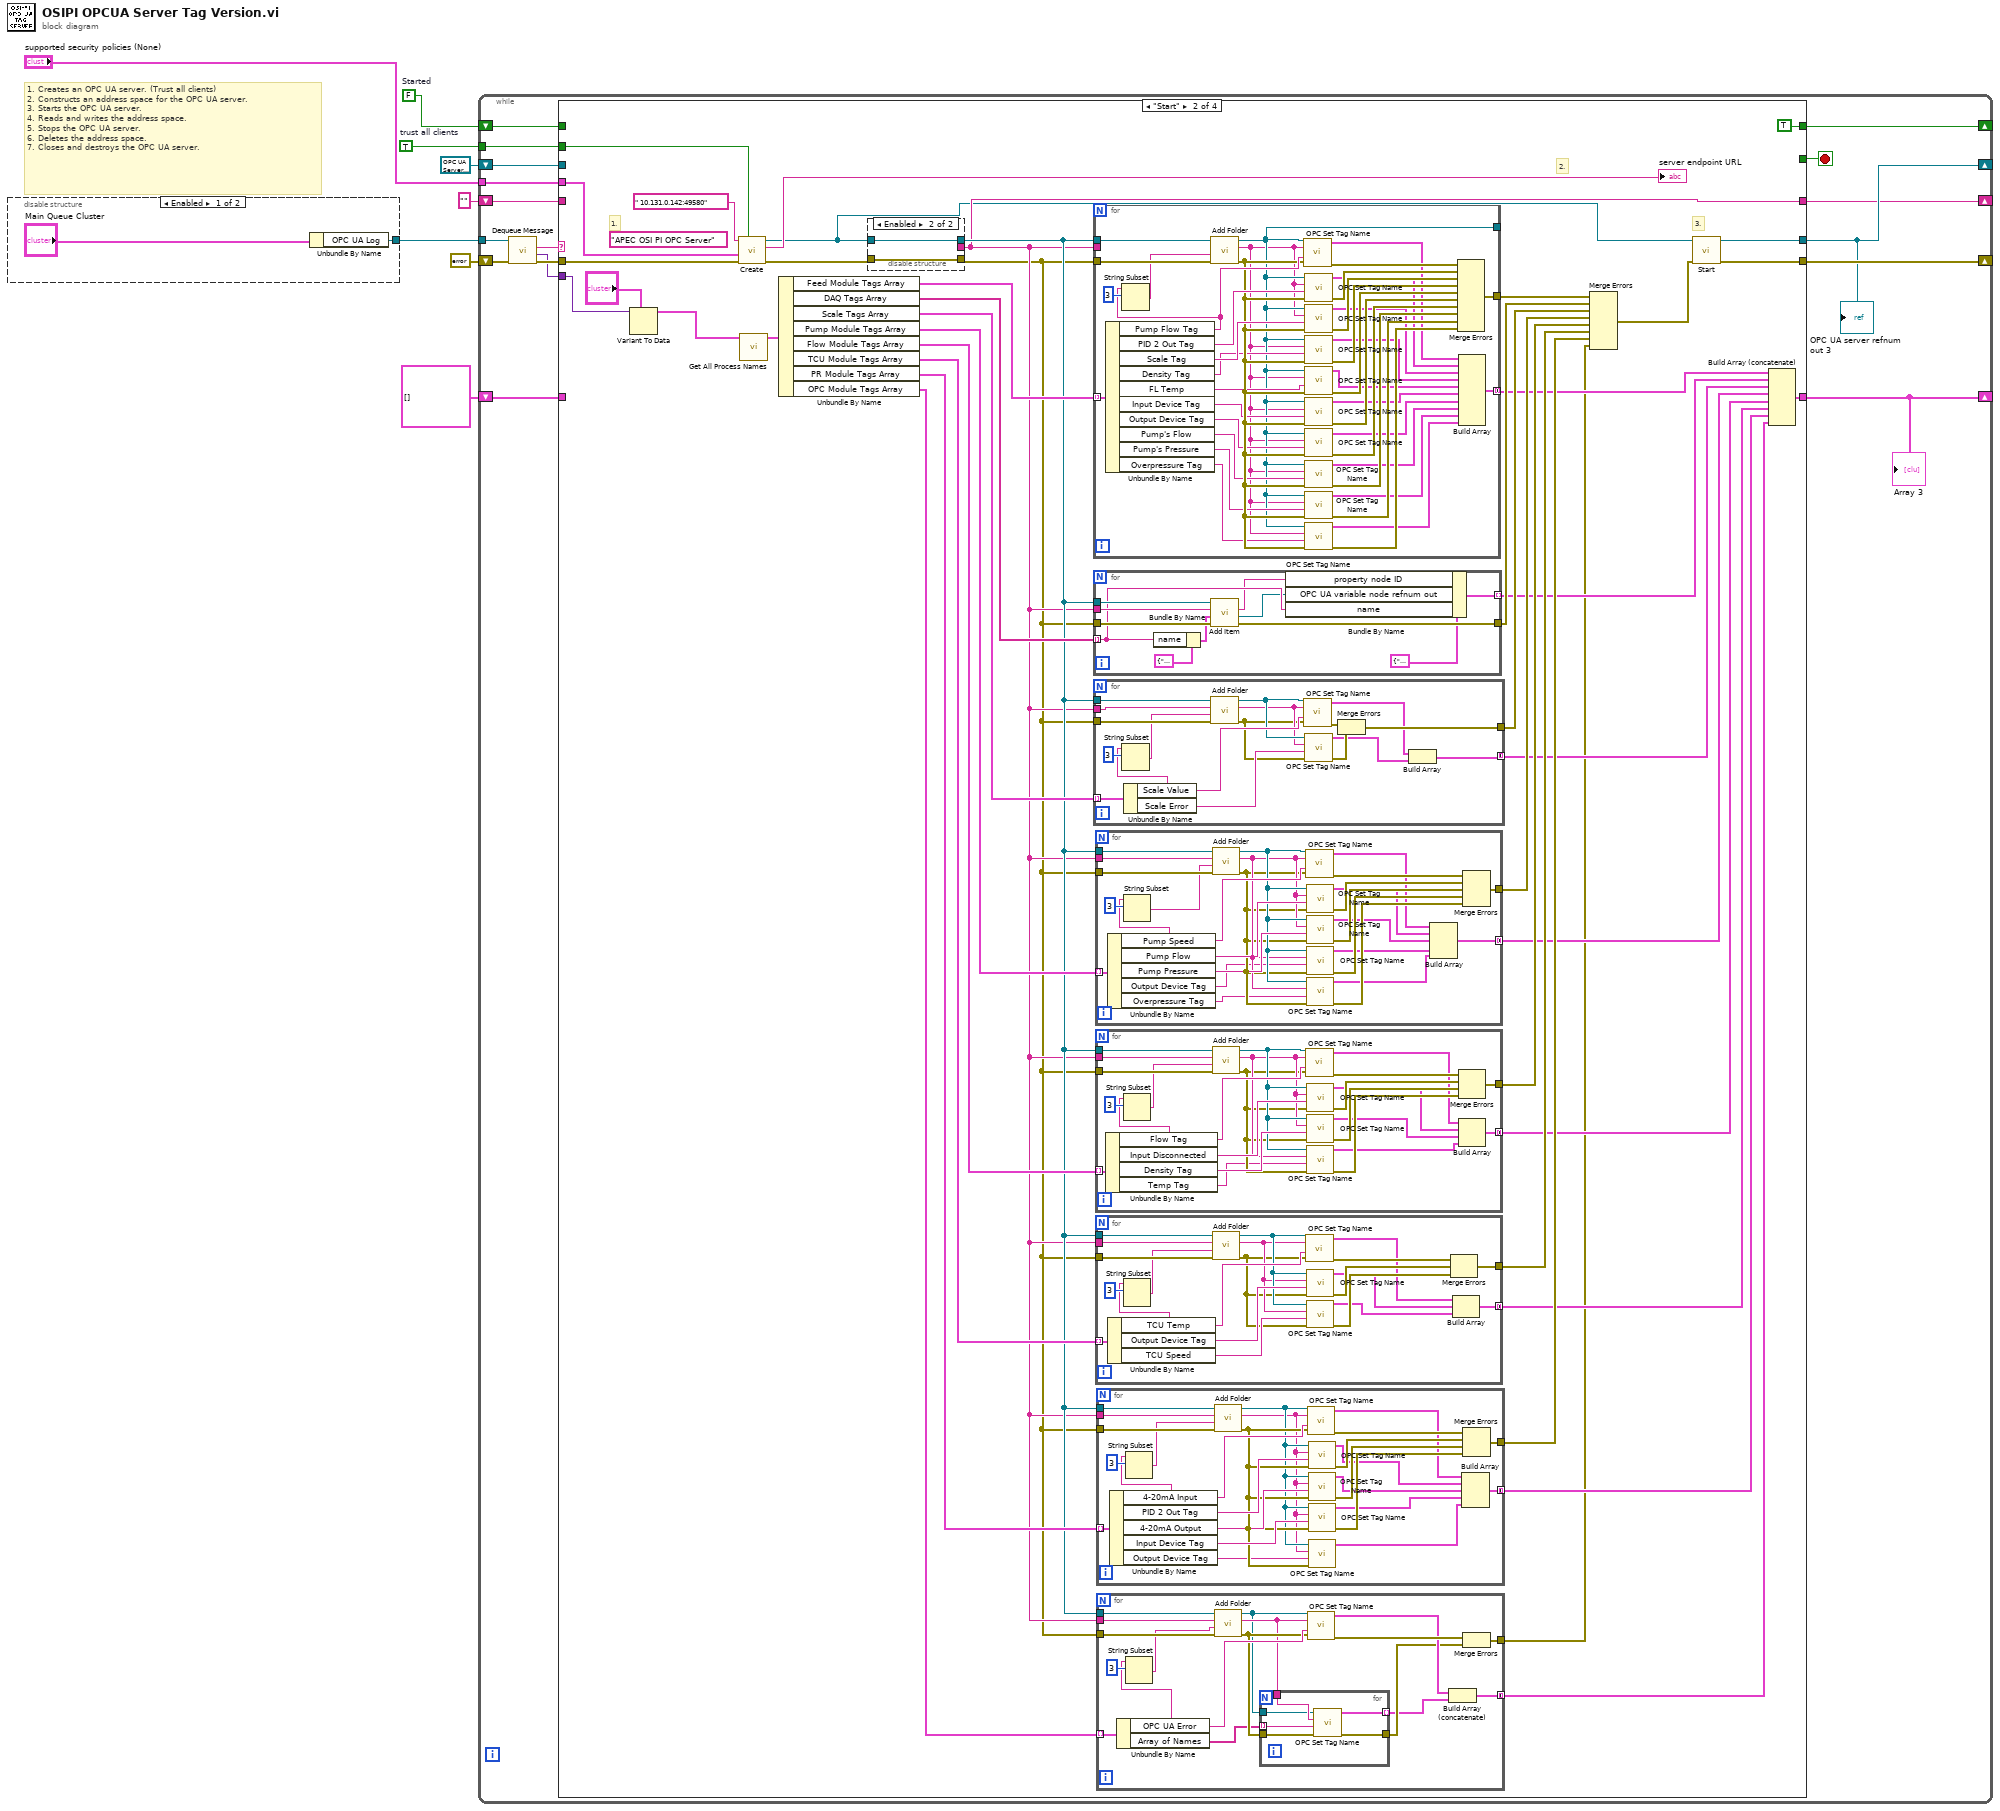
[diagram p0: block diagram]
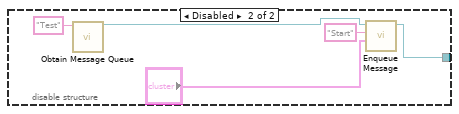
[diagram p2: hidden frame]
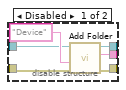
[diagram p4: hidden frame]
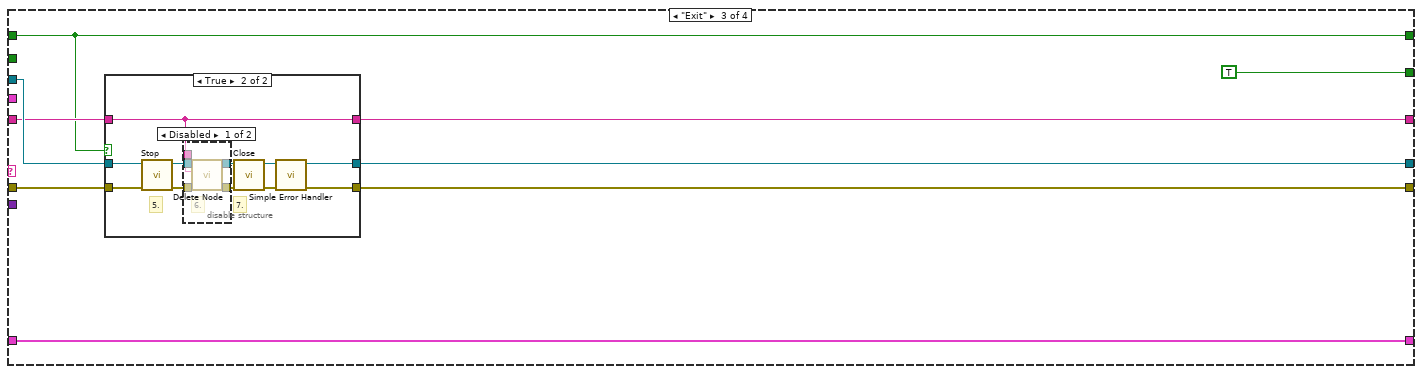
[diagram p5: hidden frame]
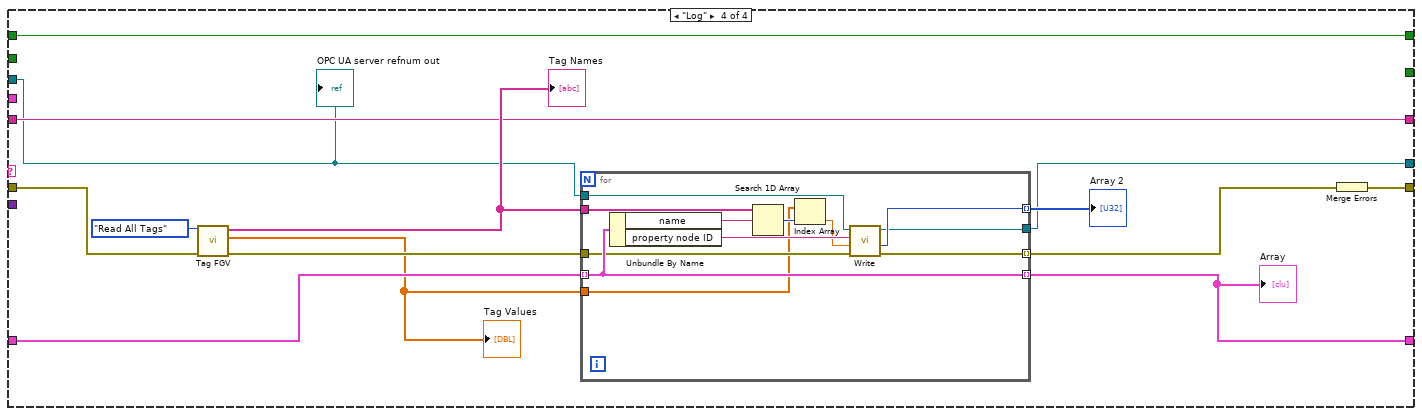
[diagram p8: hidden frame]
diagram:
  w1 = FALSE  # Started
  w8 = TRUE  # trust all clients
  # "1. Creates an OPC UA server. (Trust all clients)\n2. Constructs an address space for the OPC UA server.\n3. Starts the OPC UA server.\n4. Reads and writes the address space.\n5. Stops the OPC UA server.\n6. Deletes the address space.\n7. Closes and destroys the OPC UA server."
  n1 = disable-structure shown="Enabled" {
    disable-tunnel: [w9 w12] -> w6
    frame Enabled {
      n2 = Unbundle By Name("Main Queue Cluster") -> ("OPC UA Log"=w9:refnum<queue>)
    }
    frame Disabled {
      n3 = call "Obtain Message Queue.vi"("name (unnamed)"="Test") -> ("Message Queue"=w11:refnum<queue>)  [unwired: 9 in, 1 out]
      n4 = call-poly "Enqueue Message.vi"("Message Data"="?", "Message"="Start", "Message Queue"=w11) -> ("dup Message Queue"=w12:refnum<queue>)  [unwired: 7 in, 1 out]
    }
  }
  n5 = while {
    tunnel: w6 -> [w31]
    shift-right: [w28] -> _
    shift-left: errorcluster {"status"=FALSE, "code"=0, "source"=""} ("error IO") -> [w27]
    tunnel: w8 -> [w26]
    tunnel: "supported security policies (None)" -> [w25]
    shift-right: [w24] -> _
    shift-left: T66 refnum ("OPC UA server refnum out") -> [w23]
    shift-right: [w22] -> _
    shift-left: T13 "" ("folder node ID") -> [w20]
    shift-right: [w19] -> _
    shift-left: T65 [] -> [w18]
    shift-right: [w17] -> _
    shift-left: w1 -> [w16]
    stop <- w30 stop-if-true
    n6 = call "Dequeue Message.vi"("error in (no error)"=w27, "Message Queue"=w31) -> ("error out"=w29:errorcluster, "Message Data"=w21:variant, "Message"=w32:string)  [unwired: 6 in, 1 out]
    n7 = case shown="\"Start\"" w32 {
      tunnel: [_ _ TRUE _] -> w30
      tunnel: w29 -> [w35 w77 w281 w312]
      tunnel: [w35 w75 w280 w306] -> w28
      tunnel: w26 -> [_ w79 _ _]
      tunnel: w25 -> [_ w78 _ _]
      tunnel: [w36 w76 w278 w303] -> w24
      tunnel: w23 -> [w36 _ w279 w308]
      tunnel: [w37 w43 w274 w313] -> w22
      tunnel: w21 -> [_ w73 _ _]
      tunnel: w20 -> [w37 _ w277 w313]
      tunnel: [w34 w49 w276 w309] -> w19
      tunnel: w18 -> [w34 _ w276 w310]
      tunnel: w16 -> [w33 _ w275 w302]
      tunnel: [w33 TRUE ("Started") w275 w302] -> w17
      frame Default {
      }
      frame "Start" {
        (unwired) "APEC OSI PI OPC Server" ("OPC UA server name")
        # "3."
        # "2."
        # "1."
        n8 = Variant To Data(type="?", Variant=w73) -> (data=w71:T1)  [unwired: 1 in, 1 out]
        n9 = call <vilib>:"Create.vi"("trust all clients (F)"=w79, "error in (no error)"=w77, "supported security policies (None)"=w78, "OPC UA server name"=" 10.131.0.142:49580") -> ("error out"=w74:errorcluster, "server endpoint URL"=→"server endpoint URL":string, "OPC UA server refnum out"=w40:T66)  [unwired: 5 in]
        n10 = call "Get All Process Names.vi"(11:w71) -> ("Module Tags Array Cluster"=w69:T76)  [unwired: 10 in]
        n11 = Unbundle By Name(w69) -> ("Feed Module Tags Array"=w70:T71[], "DAQ Tags Array"=w68:string[], "Scale Tags Array"=w64:T77, "Pump Module Tags Array"=w62:T72[], "Flow Module Tags Array"=w60:T73[], "TCU Module Tags Array"=w58:T74[], "PR Module Tags Array"=w57:T75[], "OPC Module Tags Array"=w41:T78)
        n12 = disable-structure shown="Enabled" {
          disable-tunnel: w74 -> [w86 w87]
          disable-tunnel: [w84 w88] -> w44
          disable-tunnel: [w83 _] -> w43
          disable-tunnel: [w82 w87] -> w42
          disable-tunnel: w40 -> [w81 w88]
          frame Disabled {
            n13 = call <vilib>:"Add Folder.vi"("error in (no error)"=w86, "folder name"="Device", "OPC UA server refnum in"=w81) -> ("error out"=w82:errorcluster, "folder node ID"=w83:T13, "OPC UA server refnum out"=w84:T66)  [unwired: 5 in]
          }
          frame Enabled {
          }
        }
        n14 = for {
          tunnel: w42 -> [w273]
          tunnel: w43 -> [_]
          tunnel: w44 -> [w272]
          tunnel: [w269] -> w66
          tunnel: [w235] -> _
          tunnel: w70 -> [w271] mode=indexing
          tunnel: [w237] -> w54 mode=concatenating
          n15 = Unbundle By Name(w271) -> ("Pump Flow Tag"=w267:string, "PID 2 Out Tag"=w266:string, "Scale Tag"=w268:string, "Density Tag"=w261:string, "FL Temp"=w260:string, "Input Device Tag"=w259:string, "Output Device Tag"=w258:string, "Pump's Flow"=w257:string, "Pump's Pressure"=w256:string, "Overpressure Tag"=w255:string)
          n16 = String Subset(string=w267, length (rest)=3 ("length (rest)")) -> (substring=w236:string)  [unwired: 1 in]
          n17 = call <vilib>:"Add Folder.vi"("error in (no error)"=w273, "folder name"=w236, "OPC UA server refnum in"=w272) -> ("error out"=w262:errorcluster, "folder node ID"=w234:T13, "OPC UA server refnum out"=w235:T66)  [unwired: 5 in]
          n18 = call "OPC Set Tag Name.vi"("error in (no error)"=w262, "name"=w267, "item node ID"=w234, "Refnum in"=w235) -> ("error out"=w265:errorcluster, "OPC Property cluster"=w247:T67)  [unwired: 6 in]
          n19 = call "OPC Set Tag Name.vi"("error in (no error)"=w262, "name"=w266, "item node ID"=w234, "Refnum in"=w235) -> ("error out"=w264:errorcluster, "OPC Property cluster"=w246:T67)  [unwired: 6 in]
          n20 = call "OPC Set Tag Name.vi"("error in (no error)"=w262, "name"=w268, "item node ID"=w234, "Refnum in"=w235) -> ("error out"=w263:errorcluster, "OPC Property cluster"=w245:T67)  [unwired: 6 in]
          n21 = call "OPC Set Tag Name.vi"("error in (no error)"=w262, "name"=w261, "item node ID"=w234, "Refnum in"=w235) -> ("error out"=w254:errorcluster, "OPC Property cluster"=w244:T67)  [unwired: 6 in]
          n22 = call "OPC Set Tag Name.vi"("error in (no error)"=w262, "name"=w260, "item node ID"=w234, "Refnum in"=w235) -> ("error out"=w253:errorcluster, "OPC Property cluster"=w243:T67)  [unwired: 6 in]
          n23 = call "OPC Set Tag Name.vi"("error in (no error)"=w262, "name"=w259, "item node ID"=w234, "Refnum in"=w235) -> ("error out"=w252:errorcluster, "OPC Property cluster"=w242:T67)  [unwired: 6 in]
          n24 = call "OPC Set Tag Name.vi"("error in (no error)"=w262, "name"=w258, "item node ID"=w234, "Refnum in"=w235) -> ("error out"=w251:errorcluster, "OPC Property cluster"=w241:T67)  [unwired: 6 in]
          n25 = call "OPC Set Tag Name.vi"("error in (no error)"=w262, "name"=w257, "item node ID"=w234, "Refnum in"=w235) -> ("error out"=w250:errorcluster, "OPC Property cluster"=w240:T67)  [unwired: 6 in]
          n26 = call "OPC Set Tag Name.vi"("error in (no error)"=w262, "name"=w256, "item node ID"=w234, "Refnum in"=w235) -> ("error out"=w249:errorcluster, "OPC Property cluster"=w239:T67)  [unwired: 6 in]
          n27 = call "OPC Set Tag Name.vi"("error in (no error)"=w262, "name"=w255, "item node ID"=w234, "Refnum in"=w235) -> ("error out"=w248:errorcluster, "OPC Property cluster"=w238:T67)  [unwired: 6 in]
          n28 = Merge Errors(w265, w264, w263, w254, w253, w252, w251, w250, w249, w248) -> (w269:errorcluster)
          n29 = Build Array(w247, w246, w245, w244, w243, w242, w241, w240, w239, w238) -> (w237:T65)
        }
        n30 = for {
          tunnel: w42 -> [w233]
          tunnel: w43 -> [w232]
          tunnel: w44 -> [w231]
          tunnel: [w228] -> w67
          tunnel: w68 -> [w226] mode=indexing
          tunnel: [w223] -> w53 mode=indexing
          n31 = Bundle By Name(cluster=T69 {"name"="Node", "data type"=11, "access level"=3, "description"=""} ("item"), "name"=w226) -> (w229:T69)
          n32 = call <vilib>:"Add Item.vi"("error in (no error)"=w233, "item"=w229, "parent folder node ID"=w232, "OPC UA server refnum in"=w231) -> ("error out"=w228:errorcluster, "OPC UA variable node refnum out"=w225:T64, "item node ID"=w224:T13)  [unwired: 3 in, 1 out]
          n33 = Bundle By Name(cluster=T67 {"property node ID"="", "OPC UA variable node refnum out"="", "name"=""} ("OPC Property cluster"), "property node ID"=w224, "OPC UA variable node refnum out"=w225, "name"=w226) -> (w223:T67)
        }
        n34 = for {
          tunnel: [w220] -> w63
          tunnel: w64 -> [w222] mode=indexing
          tunnel: w44 -> [w212]
          tunnel: w43 -> [w211]
          tunnel: w42 -> [w210]
          tunnel: [w207] -> w52 mode=concatenating
          n35 = Unbundle By Name(w222) -> ("Scale Value"=w219:string, "Scale Error"=w218:string)
          n36 = String Subset(string=w219, length (rest)=3 ("length (rest)")) -> (substring=w206:string)  [unwired: 1 in]
          n37 = call <vilib>:"Add Folder.vi"("error in (no error)"=w210, "folder name"=w206, "parent folder node ID"=w211, "OPC UA server refnum in"=w212) -> ("error out"=w213:errorcluster, "folder node ID"=w214:T13, "OPC UA server refnum out"=w215:T66)  [unwired: 4 in]
          n38 = call "OPC Set Tag Name.vi"("error in (no error)"=w213, "name"=w219, "item node ID"=w214, "Refnum in"=w215) -> ("error out"=w217:errorcluster, "OPC Property cluster"=w209:T67)  [unwired: 6 in]
          n39 = call "OPC Set Tag Name.vi"("error in (no error)"=w213, "name"=w218, "item node ID"=w214, "Refnum in"=w215) -> ("error out"=w216:errorcluster, "OPC Property cluster"=w208:T67)  [unwired: 6 in]
          n40 = Merge Errors(w217, w216) -> (w220:errorcluster)
          n41 = Build Array(w209, w208) -> (w207:T65)
        }
        n42 = for {
          tunnel: w42 -> [w205]
          tunnel: w43 -> [w204]
          tunnel: w44 -> [w203]
          tunnel: [w200] -> w61
          tunnel: w62 -> [w202] mode=indexing
          tunnel: [w181] -> w51 mode=concatenating
          n43 = Unbundle By Name(w202) -> ("Pump Speed"=w198:string, "Pump Flow"=w197:string, "Pump Pressure"=w199:string, "Output Device Tag"=w190:string, "Overpressure Tag"=w189:string)
          n44 = String Subset(string=w198, length (rest)=3 ("length (rest)")) -> (substring=w180:string)  [unwired: 1 in]
          n45 = call <vilib>:"Add Folder.vi"("error in (no error)"=w205, "folder name"=w180, "parent folder node ID"=w204, "OPC UA server refnum in"=w203) -> ("error out"=w191:errorcluster, "folder node ID"=w192:T13, "OPC UA server refnum out"=w193:T66)  [unwired: 4 in]
          n46 = call "OPC Set Tag Name.vi"("error in (no error)"=w191, "name"=w198, "item node ID"=w192, "Refnum in"=w193) -> ("error out"=w196:errorcluster, "OPC Property cluster"=w186:T67)  [unwired: 6 in]
          n47 = call "OPC Set Tag Name.vi"("error in (no error)"=w191, "name"=w197, "item node ID"=w192, "Refnum in"=w193) -> ("error out"=w195:errorcluster, "OPC Property cluster"=w185:T67)  [unwired: 6 in]
          n48 = call "OPC Set Tag Name.vi"("error in (no error)"=w191, "name"=w199, "item node ID"=w192, "Refnum in"=w193) -> ("error out"=w194:errorcluster, "OPC Property cluster"=w184:T67)  [unwired: 6 in]
          n49 = call "OPC Set Tag Name.vi"("error in (no error)"=w191, "name"=w190, "item node ID"=w192, "Refnum in"=w193) -> ("error out"=w188:errorcluster, "OPC Property cluster"=w183:T67)  [unwired: 6 in]
          n50 = call "OPC Set Tag Name.vi"("error in (no error)"=w191, "name"=w189, "item node ID"=w192, "Refnum in"=w193) -> ("error out"=w187:errorcluster, "OPC Property cluster"=w182:T67)  [unwired: 6 in]
          n51 = Build Array(w186, w185, w184, w183, w182) -> (w181:T65)
          n52 = Merge Errors(w196, w195, w194, w188, w187) -> (w200:errorcluster)
        }
        n53 = for {
          tunnel: w42 -> [w179]
          tunnel: w43 -> [w178]
          tunnel: w44 -> [w177]
          tunnel: [w174] -> w59
          tunnel: w60 -> [w176] mode=indexing
          tunnel: [w158] -> w50 mode=concatenating
          n54 = Unbundle By Name(w176) -> ("Flow Tag"=w172:string, "Input Disconnected"=w171:string, "Density Tag"=w173:string, "Temp Tag"=w164:string)
          n55 = String Subset(string=w172, length (rest)=3 ("length (rest)")) -> (substring=w157:string)  [unwired: 1 in]
          n56 = call <vilib>:"Add Folder.vi"("error in (no error)"=w179, "folder name"=w157, "parent folder node ID"=w178, "OPC UA server refnum in"=w177) -> ("error out"=w165:errorcluster, "folder node ID"=w166:T13, "OPC UA server refnum out"=w167:T66)  [unwired: 4 in]
          n57 = call "OPC Set Tag Name.vi"("error in (no error)"=w165, "name"=w172, "item node ID"=w166, "Refnum in"=w167) -> ("error out"=w170:errorcluster, "OPC Property cluster"=w162:T67)  [unwired: 6 in]
          n58 = call "OPC Set Tag Name.vi"("error in (no error)"=w165, "name"=w171, "item node ID"=w166, "Refnum in"=w167) -> ("error out"=w169:errorcluster, "OPC Property cluster"=w161:T67)  [unwired: 6 in]
          n59 = call "OPC Set Tag Name.vi"("error in (no error)"=w165, "name"=w173, "item node ID"=w166, "Refnum in"=w167) -> ("error out"=w168:errorcluster, "OPC Property cluster"=w160:T67)  [unwired: 6 in]
          n60 = call "OPC Set Tag Name.vi"("error in (no error)"=w165, "name"=w164, "item node ID"=w166, "Refnum in"=w167) -> ("error out"=w163:errorcluster, "OPC Property cluster"=w159:T67)  [unwired: 6 in]
          n61 = Merge Errors(w170, w169, w168, w163) -> (w174:errorcluster)
          n62 = Build Array(w162, w161, w160, w159) -> (w158:T65)
        }
        n63 = for {
          tunnel: w42 -> [w156]
          tunnel: w43 -> [w155]
          tunnel: w44 -> [w154]
          tunnel: [w151] -> w56
          tunnel: w58 -> [w153] mode=indexing
          tunnel: [w138] -> w48 mode=concatenating
          n64 = Unbundle By Name(w153) -> ("TCU Temp"=w149:string, "Output Device Tag"=w148:string, "TCU Speed"=w150:string)
          n65 = String Subset(string=w149, length (rest)=3 ("length (rest)")) -> (substring=w137:string)  [unwired: 1 in]
          n66 = call <vilib>:"Add Folder.vi"("error in (no error)"=w156, "folder name"=w137, "parent folder node ID"=w155, "OPC UA server refnum in"=w154) -> ("error out"=w142:errorcluster, "folder node ID"=w143:T13, "OPC UA server refnum out"=w144:T66)  [unwired: 4 in]
          n67 = call "OPC Set Tag Name.vi"("error in (no error)"=w142, "name"=w149, "item node ID"=w143, "Refnum in"=w144) -> ("error out"=w147:errorcluster, "OPC Property cluster"=w141:T67)  [unwired: 6 in]
          n68 = call "OPC Set Tag Name.vi"("error in (no error)"=w142, "name"=w148, "item node ID"=w143, "Refnum in"=w144) -> ("error out"=w146:errorcluster, "OPC Property cluster"=w140:T67)  [unwired: 6 in]
          n69 = call "OPC Set Tag Name.vi"("error in (no error)"=w142, "name"=w150, "item node ID"=w143, "Refnum in"=w144) -> ("error out"=w145:errorcluster, "OPC Property cluster"=w139:T67)  [unwired: 6 in]
          n70 = Merge Errors(w147, w146, w145) -> (w151:errorcluster)
          n71 = Build Array(w141, w140, w139) -> (w138:T65)
        }
        n72 = for {
          tunnel: w42 -> [w136]
          tunnel: w43 -> [w135]
          tunnel: w44 -> [w134]
          tunnel: [w131] -> w55
          tunnel: w57 -> [w133] mode=indexing
          tunnel: [w113] -> w47 mode=concatenating
          n73 = Unbundle By Name(w133) -> ("4-20mA Input"=w129:string, "PID 2 Out Tag"=w128:string, "4-20mA Output"=w130:string, "Input Device Tag"=w123:string, "Output Device Tag"=w119:string)
          n74 = String Subset(string=w129, length (rest)=3 ("length (rest)")) -> (substring=w112:string)  [unwired: 1 in]
          n75 = call <vilib>:"Add Folder.vi"("error in (no error)"=w136, "folder name"=w112, "parent folder node ID"=w135, "OPC UA server refnum in"=w134) -> ("error out"=w122:errorcluster, "folder node ID"=w120:T13, "OPC UA server refnum out"=w121:T66)  [unwired: 4 in]
          n76 = call "OPC Set Tag Name.vi"("error in (no error)"=w122, "name"=w129, "item node ID"=w120, "Refnum in"=w121) -> ("error out"=w127:errorcluster, "OPC Property cluster"=w118:T67)  [unwired: 6 in]
          n77 = call "OPC Set Tag Name.vi"("error in (no error)"=w122, "name"=w128, "item node ID"=w120, "Refnum in"=w121) -> ("error out"=w126:errorcluster, "OPC Property cluster"=w117:T67)  [unwired: 6 in]
          n78 = call "OPC Set Tag Name.vi"("error in (no error)"=w122, "name"=w130, "item node ID"=w120, "Refnum in"=w121) -> ("error out"=w125:errorcluster, "OPC Property cluster"=w116:T67)  [unwired: 6 in]
          n79 = call "OPC Set Tag Name.vi"("error in (no error)"=w122, "name"=w123, "item node ID"=w120, "Refnum in"=w121) -> ("error out"=w124:errorcluster, "OPC Property cluster"=w115:T67)  [unwired: 6 in]
          n80 = call "OPC Set Tag Name.vi"("error in (no error)"=w122, "name"=w119, "item node ID"=w120, "Refnum in"=w121) -> ("OPC Property cluster"=w114:T67)  [unwired: 6 in, 1 out]
          n81 = Build Array(w118, w117, w116, w115, w114) -> (w113:T65)
          n82 = Merge Errors(w127, w126, w125, w124) -> (w131:errorcluster)
        }
        n83 = for {
          tunnel: w42 -> [w105]
          tunnel: w43 -> [w104]
          tunnel: w44 -> [w103]
          tunnel: [w100] -> w45
          tunnel: w41 -> [w102] mode=indexing
          tunnel: [w96] -> w46 mode=concatenating
          n84 = Unbundle By Name(w102) -> ("OPC UA Error"=w99:string, "Array of Names"=w91:string[])
          n85 = String Subset(string=w99, length (rest)=3 ("length (rest)")) -> (substring=w89:string)  [unwired: 1 in]
          n86 = call <vilib>:"Add Folder.vi"("error in (no error)"=w105, "folder name"=w89, "parent folder node ID"=w104, "OPC UA server refnum in"=w103) -> ("error out"=w95:errorcluster, "folder node ID"=w94:T13, "OPC UA server refnum out"=w93:T66)  [unwired: 4 in]
          n87 = for {
            tunnel: w95 -> [w111]
            tunnel: w94 -> [w110]
            tunnel: w93 -> [w109]
            tunnel: [w108] -> w92
            tunnel: w91 -> [w107] mode=indexing
            tunnel: [w106] -> w90 mode=indexing
            n88 = call "OPC Set Tag Name.vi"("error in (no error)"=w111, "name"=w107, "item node ID"=w110, "Refnum in"=w109) -> ("error out"=w108:errorcluster, "OPC Property cluster"=w106:T67)  [unwired: 6 in]
          }
          n89 = call "OPC Set Tag Name.vi"("error in (no error)"=w95, "name"=w99, "item node ID"=w94, "Refnum in"=w93) -> ("error out"=w98:errorcluster, "OPC Property cluster"=w97:T67)  [unwired: 6 in]
          n90 = Build Array (concatenate)(w97, w90) -> (w96:T65)
          n91 = Merge Errors(w98, w92) -> (w100:errorcluster)
        }
        n92 = Merge Errors(w66, w67, w63, w61, w59, w56, w55, w45) -> (w65:errorcluster)
        n93 = call <vilib>:"Start.vi"("error in (no error)"=w65, "OPC UA server refnum in"=w40) -> ("error out"=w75:errorcluster, "OPC UA server refnum out"=w76:T66)  [unwired: 7 in, 1 out]
        n94 = Build Array (concatenate)(w54, w53, w52, w51, w50, w48, w47, w46) -> (w49:T65)
      }
      frame "Exit" {
        n95 = case shown="True" w275 {
          tunnel: w281 -> [w284 w290]
          tunnel: [w284 w289] -> w280
          tunnel: w279 -> [w285 w288]
          tunnel: [w285 w287] -> w278
          tunnel: w277 -> [w283 w286]
          tunnel: [w283 w286] -> w274
          frame False {
          }
          frame True {
            # "7."
            # "5."
            n96 = call <vilib>:"Stop.vi"("error in (no error)"=w290, "OPC UA server refnum in"=w288) -> ("error out"=w292:errorcluster, "OPC UA server refnum out"=w293:T66)  [unwired: 8 in]
            n97 = disable-structure shown="Disabled" {
              disable-tunnel: [w299 w300] -> w294
              disable-tunnel: w293 -> [w298 w301]
              disable-tunnel: w292 -> [w297 w300]
              disable-tunnel: [w296 w301] -> w287
              disable-tunnel: w286 -> [w295 _]
              frame Disabled {
                # "6."
                n98 = call <vilib>:"Delete Node.vi"("error in (no error)"=w297, "node ID"=w295, "OPC UA server refnum in"=w298) -> ("error out"=w299:errorcluster, "OPC UA server refnum out"=w296:T66)  [unwired: 7 in]
              }
              frame Enabled {
              }
            }
            n99 = call <vilib>:"Close.vi"("error in (no error)"=w294, "OPC UA server refnum in"=w287) -> ("error out"=w291:errorcluster)  [unwired: 9 in]
            n100 = call <vilib>:"Simple Error Handler.vi"("error in (no error)"=w291) -> ("error out"=w289:errorcluster)  [unwired: 4 in, 4 out]
          }
        }
      }
      frame "Log" {
        n101 = call "Tag FGV.vi"("error in (no error)"=w312, "Operation"=Tag_FGV_Operation_Enum."Read All Tags") -> ("error out"=w311:errorcluster, "Tag Values"=w305:dbl[], "Tag Names"=w314:string[])  [unwired: 4 in, 3 out]
        "Tag Values" <- w305
        "Tag Names" <- w314
        n102 = for {
          tunnel: w314 -> [w326]
          tunnel: w311 -> [w321]
          tunnel: w310 -> [w327] mode=indexing
          tunnel: [w327] -> w309 mode=indexing
          tunnel: w308 -> [w322]
          tunnel: [w320] -> w307 mode=indexing
          tunnel: w305 -> [w319]
          tunnel: [w317] -> w304 mode=indexing
          tunnel: [w316] -> w303
          n103 = Unbundle By Name(w327) -> ("name"=w325:string, "property node ID"=w323:T13)
          n104 = Search 1D Array(1D array=w326, element=w325) -> (index of element=w324:i32)  [unwired: 1 in]
          n105 = Index Array(array=w319, index=w324) -> (element=w318:dbl)
          n106 = call-poly <vilib>:"Write.vi"("error in (no error)"=w321, "value"=w318, "node ID"=w323, "OPC UA server refnum in"=w322) -> ("error out"=w320:errorcluster, "status"=w317:T14, "OPC UA server refnum out"=w316:T66)  [unwired: 5 in]
        }
        "Array" <- w309
        "Array 2" <- w304
        n107 = Merge Errors(w307) -> (w306:errorcluster)
        "OPC UA server refnum out" <- w308
      }
    }
    "OPC UA server refnum out 3" <- w24
    "Array 3" <- w19
  }
